vi "SVFA Get Spectrum Value (1 Ch).vi"(0 "spectrum":cluster{"x0":dbl, "dx":dbl, "magnitude":dbl[]} {"magnitude" format="%.2f"; "dx" format="%.2f"; "x0" format="%.2f"}, 2 "x value (1000)":dbl=1000.0 format="%.2f", 3 "coercion (nearest)":T1(ring), 4 "spectrum info":T2={"channel name"="", "description"="", "x-axis units"=0, "spectral info"={"spectrum type"=enum."Power [Magnitude^2]", "linear/dB"=enum."linear", "window"=0, "window size"=0, "FFT size"=0}, "engineering units"=0, "custom label"="", "dB reference [EU]"=0.0, "peak units"=enum."rms", "weighting filter"=0, "spectral density?"=FALSE, "unit label"="", "spectrum skewed?"=FALSE, "complimentary spectrum units"=enum."none"} {"x-axis units" items=["Time (s)"=0, "Frequency-CB (Hz)"=1, "Frequency-CPB (Hz)"=1248, "Frequency-Arbitrary (Hz)"=2357, "Quefrency (s)"=2, "Revolutions (rev)"=3, "Order"=4, "Speed (RPM)"=11, "Speed (rad/s)"=21, "Index"=65535]; "weighting filter" items=["Linear", "A-weighting", "B-weighting", "C-weighting", "ITU-R 468-4", "Dolby", "CCITT", "C-message", "Wb", "Wc", "Wd", "We", "Wf", "Wh", "Wj", "Wk", "Wm", "AES17 20 kHz lowpass", "AES17 40 kHz lowpass", "AES17 20 kHz highpass", "AES17 40 kHz highpass"]; "dB reference [EU]" format="%.2f"; "engineering units" items=["custom..."=0, "V"=1, "A"=21, "C"=30, "pC"=31, "s"=32, "-"=29, "Pa"=2, "N"=20, "g"=3, "m/s^2"=4, "m/s"=5, "m"=6, "mm/s"=12, "mm"=13, "micron/s"=14, "micron"=15, "in/s^2"=7, "in/s"=8, "in"=9, "mil/s"=10, "mil"=11, "rad/s^2"=16, "rad/s"=17, "rad"=18, "deg/s^2"=26, "deg/s"=27, "deg"=28, "RPM"=22, "cycle/s^2"=23, "Hz"=24, "cycle"=25, "strain"=19]; "spectral info"."window" items=["None "=0, "Hanning"=1, "Hamming"=2, "Blackman-Harris"=3, "Exact Blackman"=4, "Blackman"=5, "Flat Top"=6, "4 Term B-Harris "=7, "7 Term B-Harris"=8, "Low Sidelobe"=9, "Force - Exponential"=10, "Gaussian"=62]}, 5 "error in (no error)":errorcluster) -> (14 "spectrum value":dbl=nan format="%.2p", 15 "unit label":string, 16 "actual x value":dbl=nan format="%.2f", 17 "x label":string, 19 "error out":errorcluster)   [LabVIEW 2017]
doc: "Extracts the value of the spectrum at the specified frequency. Use the frequency coercion control to specify how the frequency should be coerced if it does not exactly coincide with a frequency line. This VI operates on any real-valued spectrum. Wire data to the <B>spectrum</B> input to determine the polymorphic instance to use or manually select the instance."
uses:
  <vilib>/addons/_NISVFA/_Shared subVIs/Controls/svc_Spectrum Info.ctl
  <vilib>/addons/_NISVFA/_Shared subVIs/Controls/svc_X-Axis Units.ctl
  <vilib>/addons/_NISVFA/_Shared subVIs/Controls/svc_Spectrum Type.ctl
  <vilib>/addons/_NISVFA/_Shared subVIs/Controls/svc_Engineering Units Text Ring.ctl
  <vilib>/addons/_NISVFA/_Shared subVIs/Controls/svc_Weighting Filter Text Ring.ctl
  <vilib>/addons/_NISVFA/_Shared subVIs/Controls/svc_Complimentary Spectrum Units.ctl
  <vilib>/addons/_NISVFA/_Shared subVIs/Common/svc_Get Weighting Enum and Labels.vi
  <vilib>/addons/_NISVFA/_Shared subVIs/Common/svc_Unit Label Lexical Class.vi
  <vilib>/addons/_NISVFA/_Shared subVIs/Common/svc_Engineering Units to Unit Label.vi
  <vilib>/addons/_NISVFA/_Shared subVIs/Common/svc_Format Value (DBL).vi
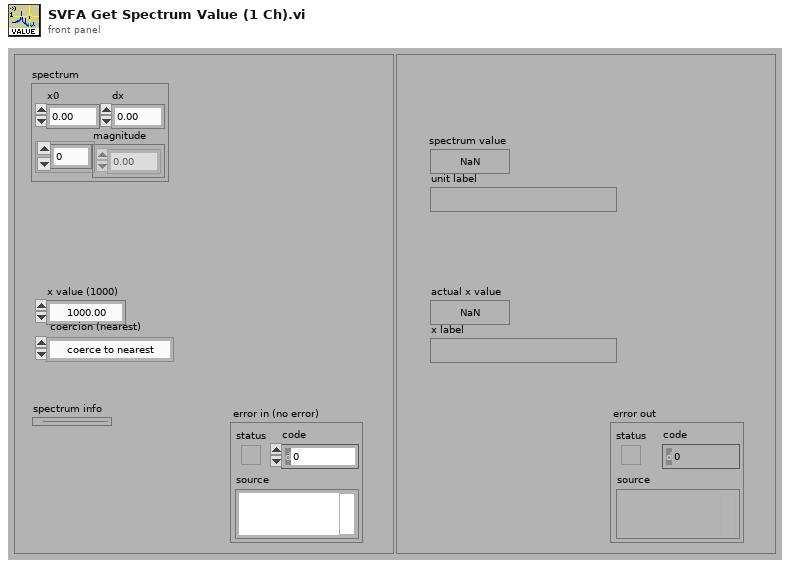
[diagram p1: front panel]
types:
  T1 = enum16{"coerce to nearest", "coerce to next highest", "coerce to next lowest", "interpolate"}
  T2 = typedef "svc_Spectrum Info.ctl" = cluster{"channel name":string, "description":string, "x-axis units":T3, "spectral info":cluster{"spectrum type":T4, "linear/dB":enum16{"linear", "dB"}, "window":u16, "window size":i32, "FFT size":i32}, "engineering units":T5, "custom label":string, "dB reference [EU]":dbl, "peak units":enum16{"rms", "peak", "peak-peak"}, "weighting filter":T6, "spectral density?":bool, "unit label":string, "spectrum skewed?":bool, "complimentary spectrum units":T7}
  T3 = typedef "svc_X-Axis Units.ctl" = u16
  T4 = typedef "svc_Spectrum Type.ctl" = enum16{"FFT Spectrum [complex]", "Amplitude [Magnitude]", "Power [Magnitude^2]", "Cross Spectrum [complex]", "Frequency Response [Complex]"}
  T5 = typedef "svc_Engineering Units Text Ring.ctl" = u16
  T6 = typedef "svc_Weighting Filter Text Ring.ctl" = u16
  T7 = typedef "svc_Complimentary Spectrum Units.ctl" = enum16{"none", "radians", "degrees", "cycles", "imaginary"}
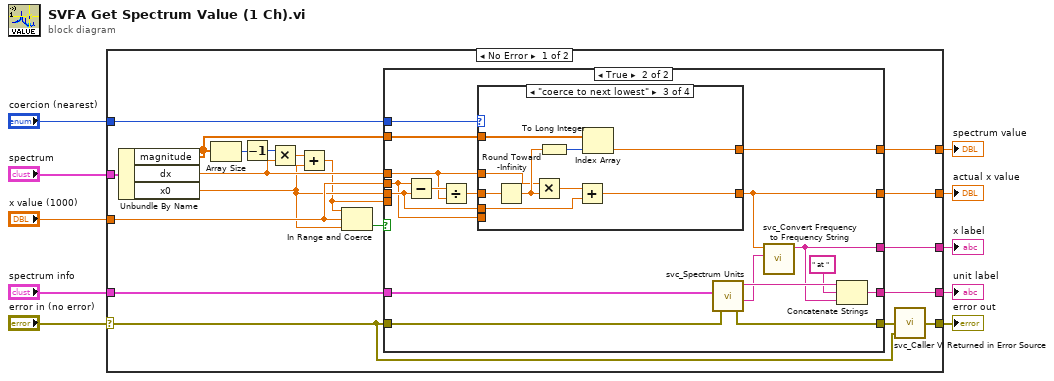
[diagram p0: block diagram]
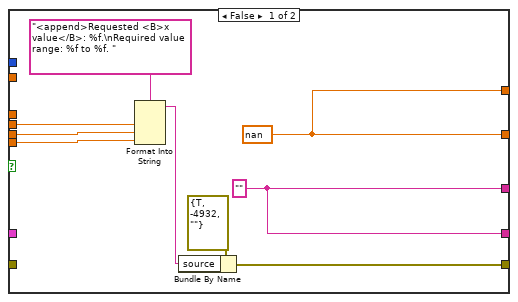
[diagram p2: hidden frame]
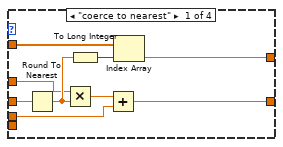
[diagram p3: hidden frame]
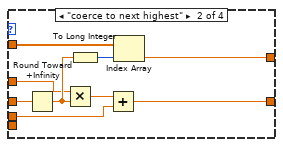
[diagram p4: hidden frame]
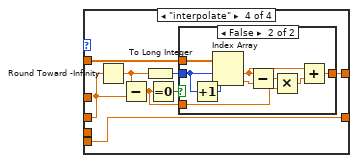
[diagram p5: hidden frame]
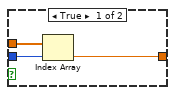
[diagram p6: hidden frame]
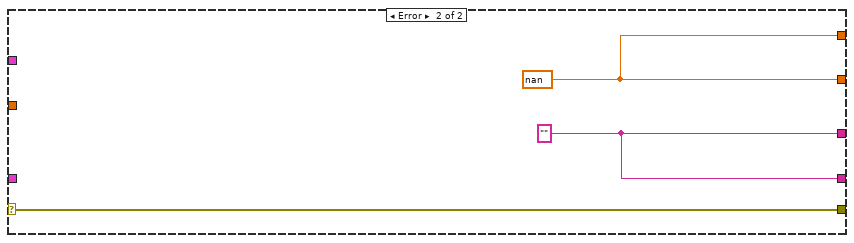
[diagram p7: hidden frame]
diagram:
  n1 = case shown="No Error" "error in (no error)" {
    selector: "error in (no error)" -> [w12 w105]
    tunnel: [w14 w105] -> w10
    tunnel: "spectrum" -> [w29 _]
    tunnel: [w27 w103] -> w8
    tunnel: "spectrum info" -> [w28 _]
    tunnel: "coercion (nearest)" -> [w21 _]
    tunnel: "x value (1000)" -> [w18 _]
    tunnel: [w24 w104] -> w4
    tunnel: [w23 w104] -> w3
    tunnel: [w20 w103] -> w2
    frame No Error {
      n2 = Unbundle By Name(w29) -> ("magnitude"=w17:dbl[], "dx"=w22:dbl, "x0"=w15:dbl)
      n3 = Array Size(array=w17) -> (size(s)=w26:i32)
      n4 = Decrement(x=w26) -> (x-1=w25:i32)
      n5 = Multiply(x=w25, y=w22) -> (x*y=w16:dbl)
      n6 = Add(x=w16, y=w15) -> (x+y=w11:dbl)
      n7 = In Range and Coerce(upper limit=w11, x=w18, lower limit=w15) -> (In Range?=w19:bool)  [unwired: 1 out]
      n8 = case shown="True" w19 {
        tunnel: w28 -> [_ w55]
        tunnel: w12 -> [_ w54]
        tunnel: [w30 w53] -> w13
        tunnel: w17 -> [_ w52]
        tunnel: [w37 w50] -> w27
        tunnel: [w38 w42] -> w24
        tunnel: [w38 w43] -> w23
        tunnel: w18 -> [w33 w41]
        tunnel: w15 -> [w32 w44]
        tunnel: w22 -> [_ w45]
        tunnel: w21 -> [_ w47]
        tunnel: [w37 w40] -> w20
        tunnel: w11 -> [w31 _]
        frame False {
          w37 = ""
          w38 = nan ("frequency [Hz]")
          n9 = Format Into String(format string="<append>Requested <B>x value</B>: %f.\nRequired value range: %f to %f. ", w33, w32, w31) -> (resulting string=w34:string)  [unwired: 2 in, 1 out]
          n10 = Bundle By Name(cluster=errorcluster {"status"=TRUE, "code"=-4932, "source"=""} ("error in (no error)"), "source"=w34) -> (w30:errorcluster)
        }
        frame True {
          n11 = Subtract(x=w41, y=w44) -> (x-y=w48:dbl)
          n12 = Divide(x=w48, y=w45) -> (x/y=w46:dbl)
          n13 = case shown="\"coerce to next lowest\"" w47 {
            tunnel: w52 -> [w64 w73 w82 w90]
            tunnel: w46 -> [w63 w72 w81 w83]
            tunnel: w45 -> [w60 w69 w78 _]
            tunnel: w44 -> [w57 w66 w75 _]
            tunnel: [w59 w68 w77 w88] -> w43
            tunnel: [w58 w67 w76 w84] -> w42
            tunnel: w41 -> [_ _ _ w84]
            frame "coerce to nearest" {
              n14 = Round To Nearest(number=w63) -> (nearest integer value=w61:dbl)
              n15 = Multiply(x=w60, y=w61) -> (x*y=w56:dbl)
              n16 = To Long Integer(number=w61) -> (32bit integer=w62:i32)
              n17 = Add(x=w56, y=w57) -> (x+y=w58:dbl)
              n18 = Index Array(array=w64, index=w62) -> (element=w59:dbl)
            }
            frame "coerce to next highest" {
              n19 = Round Toward +Infinity ("Round To +Infinity")(x=w72) -> (ceil(x): smallest int >= x=w70:dbl)
              n20 = Multiply(x=w69, y=w70) -> (x*y=w65:dbl)
              n21 = To Long Integer(number=w70) -> (32bit integer=w71:i32)
              n22 = Add(x=w65, y=w66) -> (x+y=w67:dbl)
              n23 = Index Array(array=w73, index=w71) -> (element=w68:dbl)
            }
            frame "coerce to next lowest" {
              n24 = Round Toward -Infinity ("Round To -Infinity")(1:w81) -> (0:w79:dbl)
              n25 = Multiply(x=w78, y=w79) -> (x*y=w74:dbl)
              n26 = To Long Integer(number=w79) -> (32bit integer=w80:i32)
              n27 = Add(x=w74, y=w75) -> (x+y=w76:dbl)
              n28 = Index Array(array=w82, index=w80) -> (element=w77:dbl)
            }
            frame "interpolate" {
              n29 = Round Toward -Infinity ("Round To -Infinity")(1:w83) -> (0:w87:dbl)
              n30 = Subtract(x=w87, y=w83) -> (x-y=w85:dbl)
              n31 = To Long Integer(number=w87) -> (32bit integer=w89:i32)
              n32 = Equal To 0?(x=w85) -> (x = 0?=w86:bool)
              n33 = case shown="False" w86 {
                tunnel: w90 -> [w93 w102]
                tunnel: w89 -> [w92 w100]
                tunnel: [w91 w96] -> w88
                tunnel: w85 -> [_ w98]
                frame True {
                  n34 = Index Array(array=w93, index=w92) -> (element=w91:dbl)
                }
                frame False {
                  n35 = Increment(x=w100) -> (x+1=w101:i32)
                  n36 = Index Array(array=w102, index #1=w100, index #2=w101) -> (element #1=w95:dbl, element #2=w99:dbl)
                  n37 = Subtract(x=w95, y=w99) -> (x-y=w97:dbl)
                  n38 = Multiply(x=w97, y=w98) -> (x*y=w94:dbl)
                  n39 = Add(x=w95, y=w94) -> (x+y=w96:dbl)
                }
              }
            }
          }
          n40 = call <vilib>:"svc_Spectrum Units.vi"("error in (no error)"=w54, "spectrum info in"=w55) -> ("error out"=w53:errorcluster, "x-axis unit label"=w39:string, "unit label"=w51:string)  [unwired: 2 in, 1 out]
          n41 = call <vilib>:"svc_Convert Frequency to Frequency String.vi"("x-axis unit label"=w39, "frequency [Hz]"=w42) -> ("frequency string"=w40:string)  [unwired: 9 in]
          n42 = Concatenate Strings(w51, " at " ("string"), w40) -> (w50:string)
        }
      }
      n43 = call <vilib>:"svc_Caller VI Returned in Error Source.vi"("warning input to caller"=w12, "error in (no error)"=w13) -> ("error out"=w14:errorcluster)  [unwired: 3 in]
    }
    frame Error {
      w104 = nan ("frequency [Hz]")
      w103 = "" ("frequency range string")
    }
  }
  "error out" <- w10
  "unit label" <- w8
  "actual x value" <- w4
  "spectrum value" <- w3
  "x label" <- w2
